vi "Write Helium Test Results.vi"(8 "error in (no error)":errorcluster, 10 "Fixture Name":string, 11 "Report Info":T1) -> (0 "error out":errorcluster, 3 "String":string)   [LabVIEW 2015]
uses:
  Controls/Report Config.ctl
  Tests/Controls/Test Results.ctl
  Tests/Controls/Step Result.ctl
  Tests/Controls/Startup Test.ctl
  Tests/Controls/Test Information.ctl
  Tests/Controls/Vacuum Test.ctl
  Tests/Controls/Test Timing.ctl
  Tests/Controls/Vaccum Thresholds.ctl
  Tests/Controls/Helium Test.ctl
  Tests/Controls/Helium Thresholds.ctl
  Tests/Controls/Startup Thresholds.ctl
  <userlib>/_OpenG.lib/file/file.llb/Strip Path Extension - Path__ogtk.vi
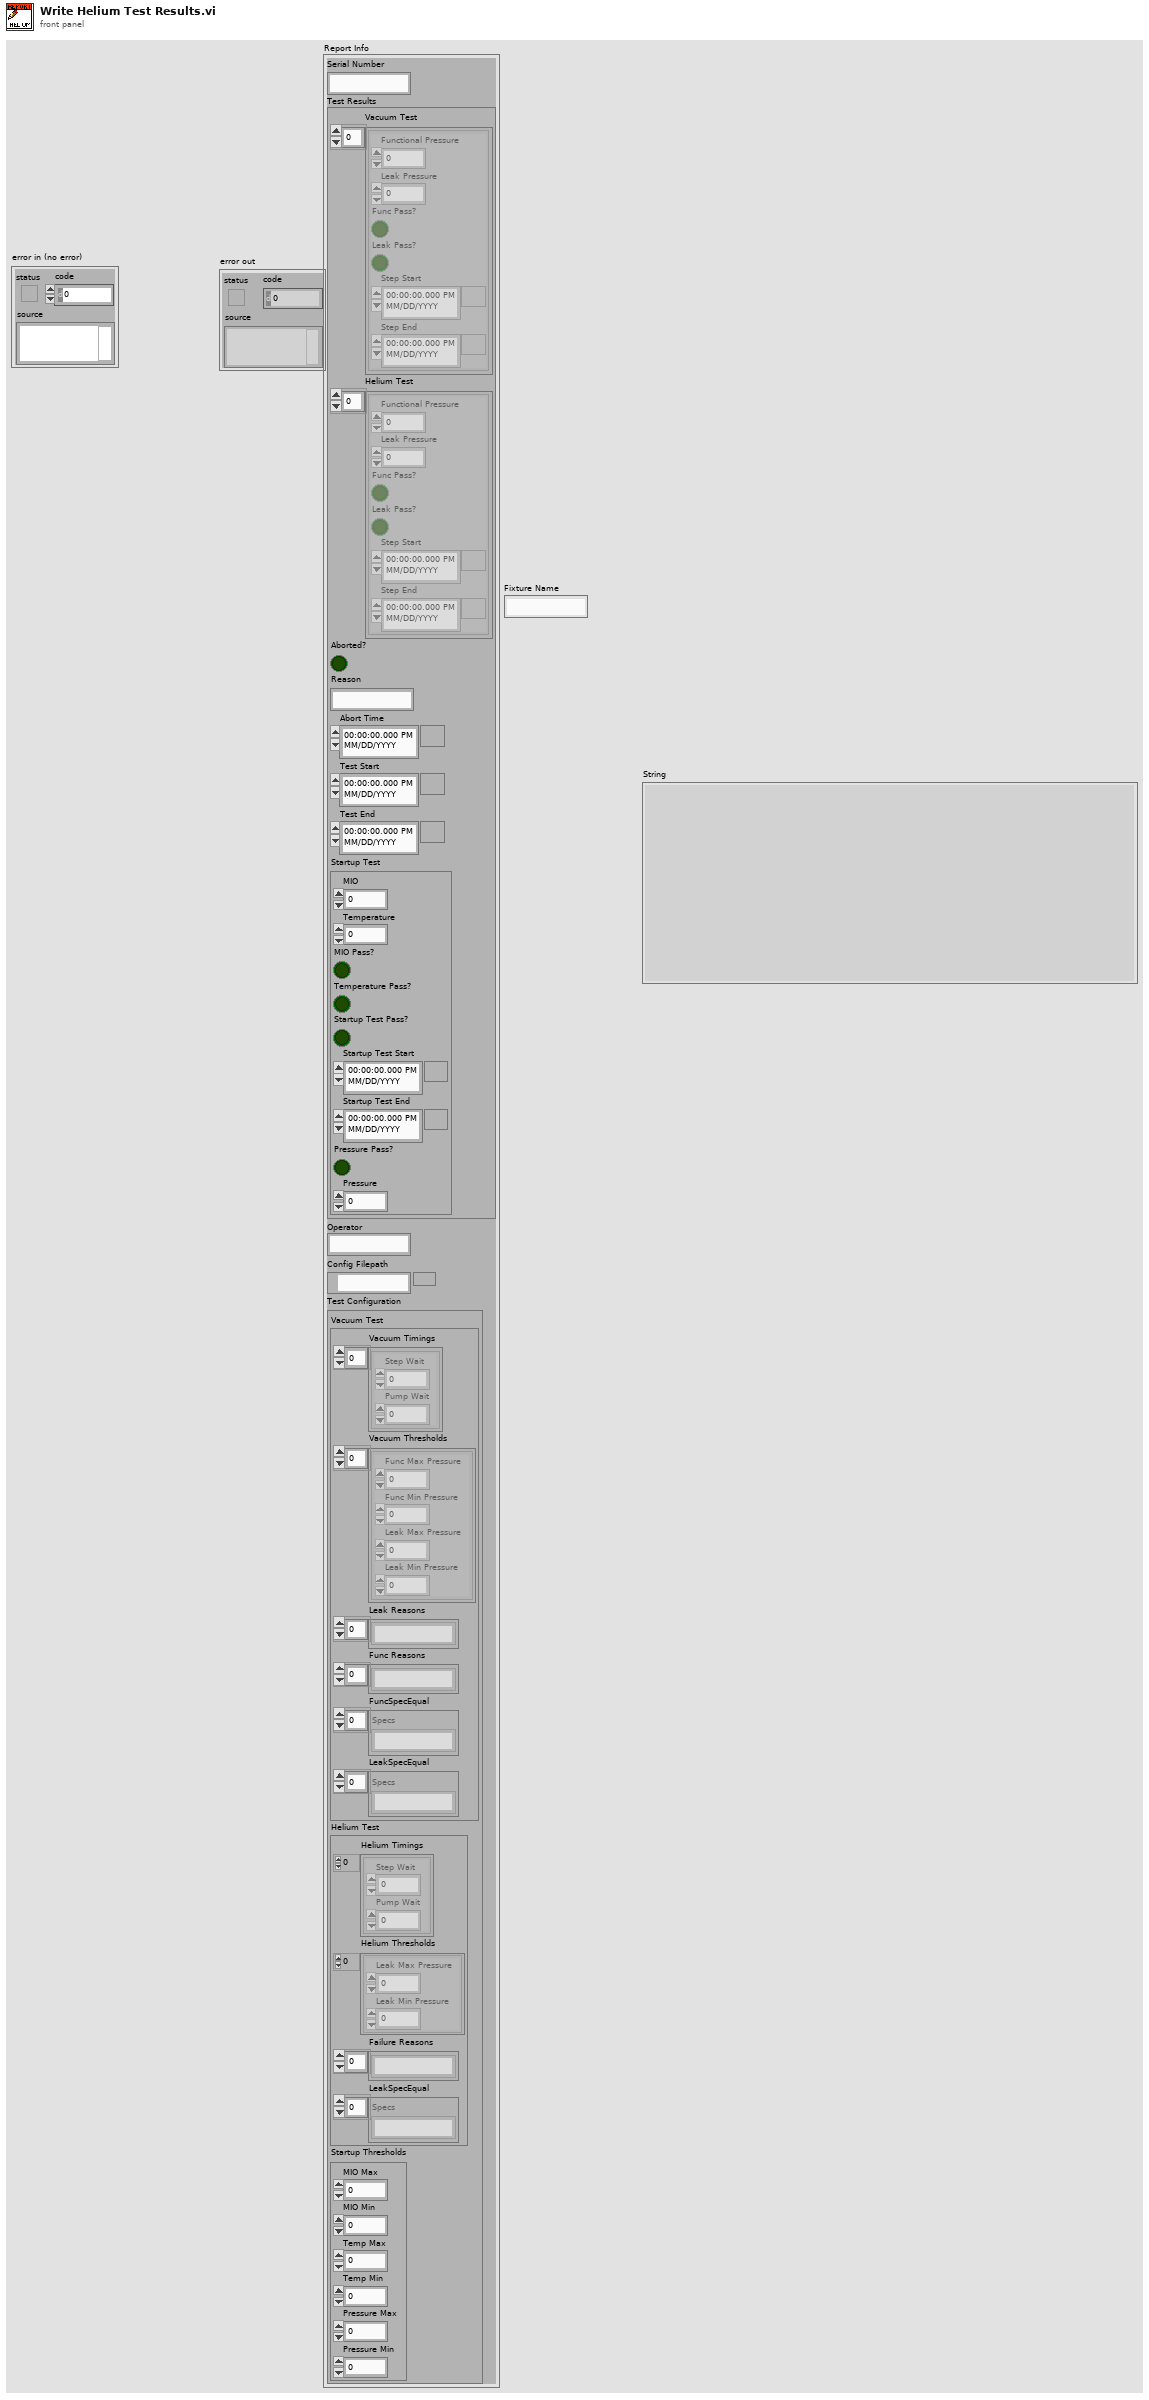
[diagram p1: front panel]
types:
  T1 = typedef "Report Config.ctl" = cluster{"Serial Number":string, "Test Results":T2, "Operator":string, "Config Filepath":path, "Test Information":T5}
  T2 = typedef "Test Results.ctl" = cluster{"Vacuum Test":T3[], "Helium Test":T3[], "Aborted?":bool, "Reason":string, "Abort Time":timestamp, "Test Start":timestamp, "Test End":timestamp, "Startup Test":T4}
  T3 = typedef "Step Result.ctl" = cluster{"Functional Pressure":dbl, "Leak Pressure":dbl, "Func Pass?":bool, "Leak Pass?":bool, "Step Start":timestamp, "Step End":timestamp}
  T4 = typedef "Startup Test.ctl" = cluster{"MIO":dbl, "Temperature":dbl, "MIO Pass?":bool, "Temperature Pass?":bool, "Startup Test Pass?":bool, "Startup Test Start":timestamp, "Startup Test End":timestamp, "Pressure Pass?":bool, "Pressure":dbl}
  T5 = typedef "Test Information.ctl" = cluster{"Vacuum Test":T6, "Helium Test":T9, "Startup Thresholds":T11}
  T6 = typedef "Vacuum Test.ctl" = cluster{"Vacuum Timings":T7[], "Vacuum Thresholds":T8[], "Leak Reasons":string[], "Func Reasons":string[], "FuncSpecEqual":string[], "LeakSpecEqual":string[]}
  T7 = typedef "Test Timing.ctl" = cluster{"Step Wait":dbl, "Pump Wait":dbl}
  T8 = typedef "Vaccum Thresholds.ctl" = cluster{"Func Max Pressure":dbl, "Func Min Pressure":dbl, "Leak Max Pressure":dbl, "Leak Min Pressure":dbl}
  T9 = typedef "Helium Test.ctl" = cluster{"Helium Timings":T7[], "Helium Thresholds":T10[], "Failure Reasons":string[], "LeakSpecEqual":string[]}
  T10 = typedef "Helium Thresholds.ctl" = cluster{"Leak Max Pressure":dbl, "Leak Min Pressure":dbl}
  T11 = typedef "Startup Thresholds.ctl" = cluster{"MIO Max":dbl, "MIO Min":dbl, "Temp Max":dbl, "Temp Min":dbl, "Pressure Max":dbl, "Pressure Min":dbl}
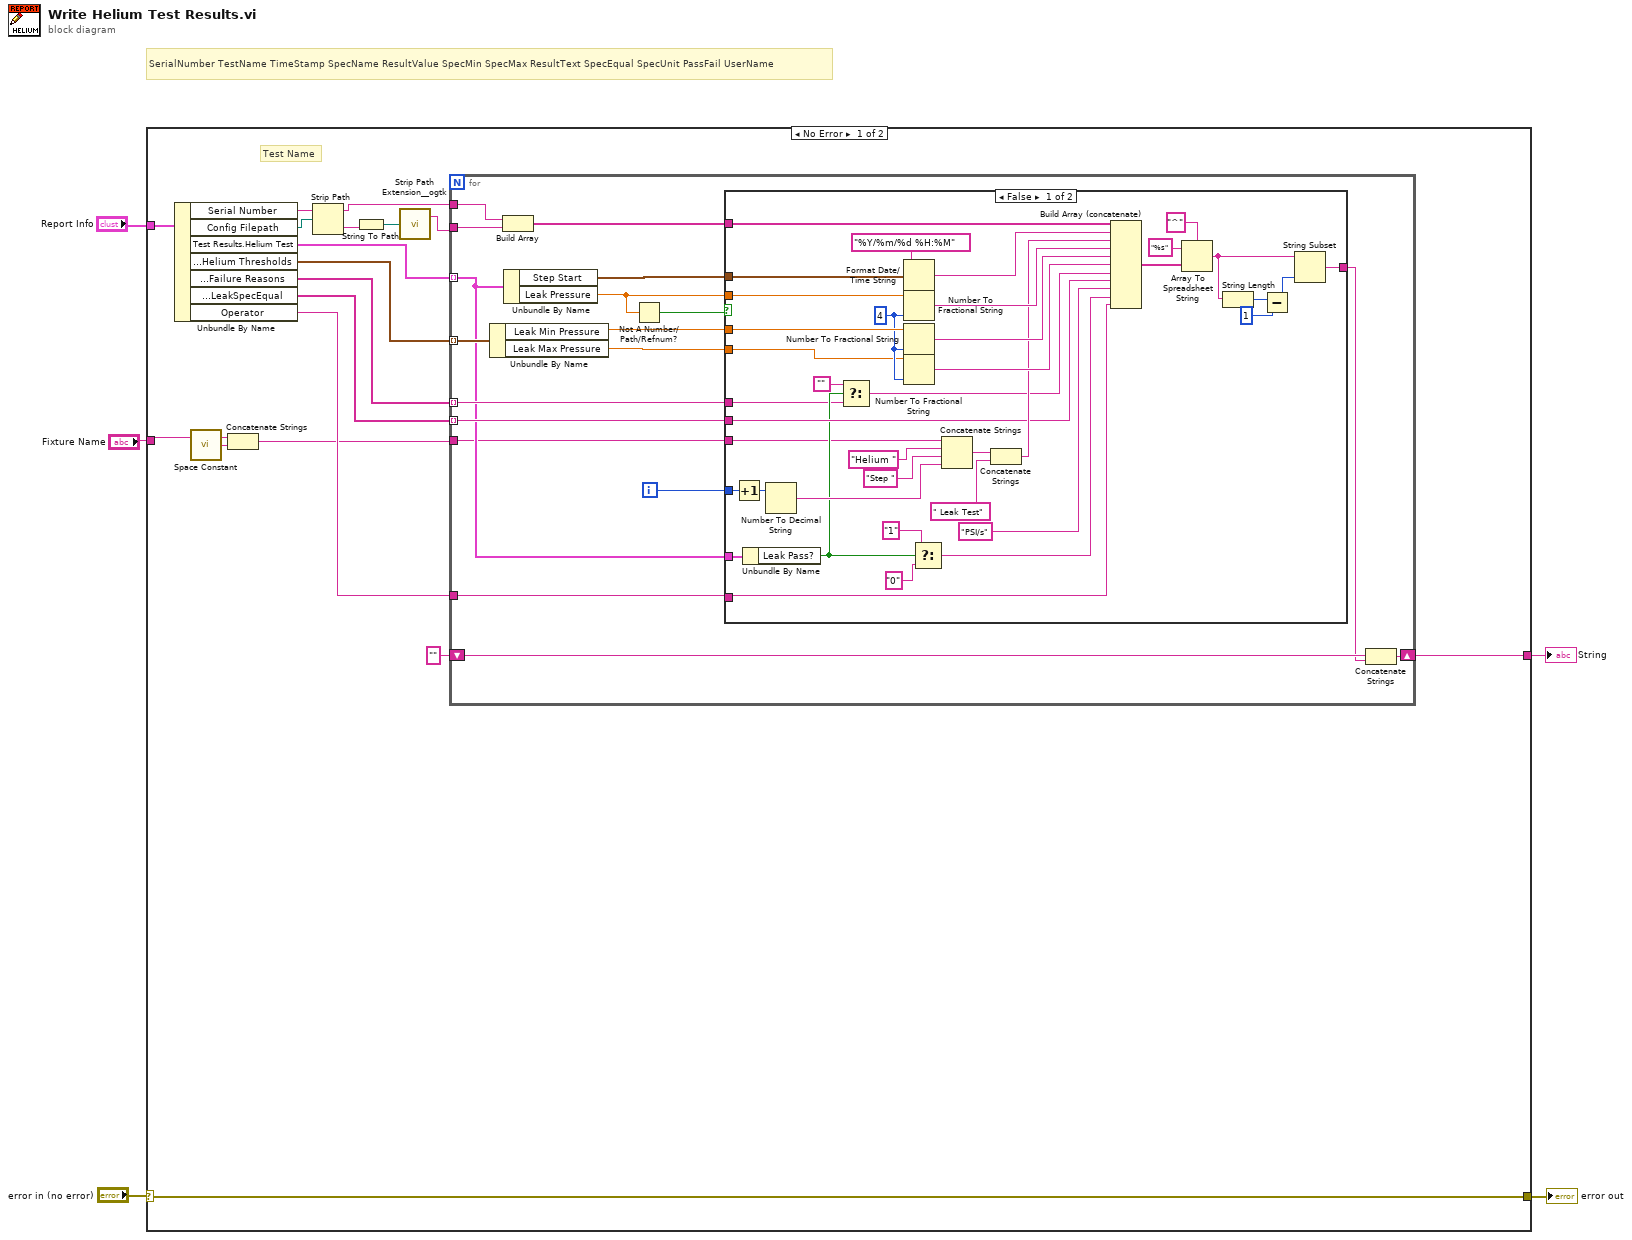
[diagram p0: block diagram]
diagram:
  # "SerialNumber\tTestName\tTimeStamp\tSpecName\tResultValue\tSpecMin\tSpecMax\tResultText\tSpecEqual\tSpecUnit\tPassFail\tUserName"
  n1 = case shown="No Error" "error in (no error)" {
    selector: "error in (no error)" -> [w10 w80]
    tunnel: [w10 w80] -> w3
    tunnel: "Report Info" -> [w22 _]
    tunnel: [w9 _] -> w2
    tunnel: "Fixture Name" -> [w7 _]
    frame No Error {
      # "Test Name"
      n2 = Unbundle By Name(w22) -> ("Serial Number"=w15:string, "Config Filepath"=w16:path, "Test Results.Helium Test"=w21:T3[], "Test Information.Helium Test.Helium Thresholds"=w20:T10[], "Test Information.Helium Test.Failure Reasons"=w19:string[], "Test Information.Vacuum Test.LeakSpecEqual"=w18:string[], "Operator"=w11:string)
      n3 = call <vilib>:"Space Constant.vi"() -> ("String"=w8:string)
      n4 = Concatenate Strings(w7, w8) -> (w6:string)
      n5 = Strip Path(path=w16) -> (name=w14:string)  [unwired: 1 out]
      n6 = String To Path(string=w14) -> (path=w12:path)
      n7 = call-poly <userlib>:"Strip Path Extension__ogtk.vi"("path"=w12) -> ("root"=w13:string)  [unwired: 1 out]
      n8 = for {
        tunnel: w21 -> [w25] mode=indexing
        tunnel: w20 -> [w27] mode=indexing
        tunnel: w19 -> [w38] mode=indexing
        tunnel: w18 -> [w37] mode=indexing
        tunnel: w11 -> [w36]
        tunnel: w15 -> [w35]
        shift-right: [w32] -> w9
        shift-left: "" -> [w31]
        tunnel: w13 -> [w30]
        tunnel: w6 -> [w23]
        i -> [w26]
        n9 = Unbundle By Name(w27) -> ("Leak Min Pressure"=w40:dbl, "Leak Max Pressure"=w39:dbl)
        n10 = Build Array(w35, w30) -> (w29:string[])
        n11 = Unbundle By Name(w25) -> ("Step Start"=w28:timestamp, "Leak Pressure"=w34:dbl)
        n12 = Not A Number/Path/Refnum?(number/path/refnum=w34) -> (NaN/Path/Refnum?=w33:bool)
        n13 = case shown="False" w33 {
          tunnel: w28 -> [w78 _]
          tunnel: w40 -> [w77 _]
          tunnel: w39 -> [w75 _]
          tunnel: w26 -> [w70 _]
          tunnel: w38 -> [w49 _]
          tunnel: w37 -> [w62 _]
          tunnel: w25 -> [w60 _]
          tunnel: w36 -> [w56 _]
          tunnel: w29 -> [w55 _]
          tunnel: w34 -> [w54 _]
          tunnel: [w45 _] -> w24
          tunnel: w23 -> [w41 _]
          frame False {
            w76 = i16 4 ("precision (6)")
            n14 = Increment(x=w70) -> (x+1=w69:i32)
            n15 = Unbundle By Name(w60) -> ("Leak Pass?"=w50:bool)
            n16 = Number To Decimal String(number=w69) -> (decimal integer string=w66:string)  [unwired: 1 in]
            n17 = Select(t="", s=w50, f=w49) -> (s? t:f=w47:string)
            n18 = Format Date/Time String(time format string (%c)="%Y/%m/%d %H:%M", seconds (now)=w78) -> (date/time string=w74:string)  [unwired: 1 in]
            n19 = Number To Fractional String(number=w54, precision (6)=w76) -> (F-format string=w73:string)  [unwired: 2 in]
            n20 = Number To Fractional String(number=w77, precision (6)=w76) -> (F-format string=w72:string)  [unwired: 2 in]
            n21 = Number To Fractional String(number=w75, precision (6)=w76) -> (F-format string=w71:string)  [unwired: 2 in]
            n22 = Select(t="1" ("string"), s=w50, f="0" ("string")) -> (s? t:f=w57:string)
            n23 = Concatenate Strings(w41, "Helium " ("string"), "Step " ("string"), w66) -> (w65:string)
            n24 = Concatenate Strings(w65, " Leak Test" ("string")) -> (w63:string)
            n25 = Build Array (concatenate)(w55, w74, w63, w73, w72, w71, w47, w62, "PSI/s" ("string"), w57, w56) -> (w53:string[])
            n26 = Array To Spreadsheet String(delimiter (Tab)="^", array=w53, 3:"%s" ("format string")) -> (spreadsheet string=w46:string)
            n27 = String Length(string=w46) -> (length=w44:i32)
            n28 = Subtract(x=w44, y=1) -> (x-y=w42:i32)
            n29 = String Subset(string=w46, length (rest)=w42) -> (substring=w45:string)  [unwired: 1 in]
          }
          frame True {
          }
        }
        n30 = Concatenate Strings(w31, w24) -> (w32:string)
      }
    }
    frame Error {
    }
  }
  "error out" <- w3
  "String" <- w2
